vi "GET Log Ref.vi"(8 "error in (no error)":errorcluster) -> (0 "error out":errorcluster, 3 "LogsAbstract out":refnum<class "LogsAbstract.lvclass">)   [LabVIEW 2019, in "LogsAbstract.lvlib" / "LogsAbstract.lvclass"]
uses:
  LogsAbstract.lvclass
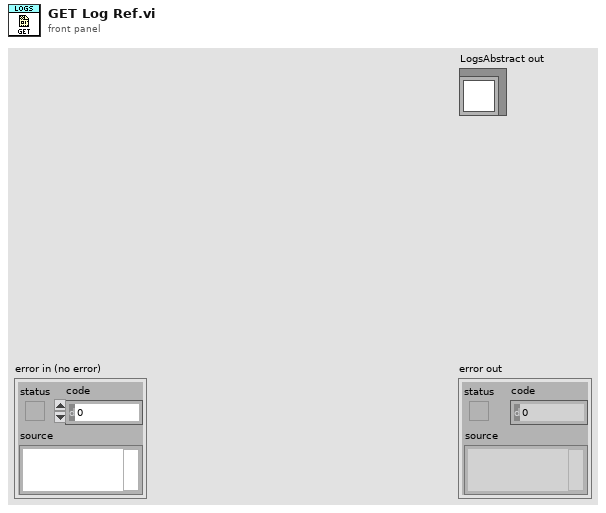
[diagram p1: front panel]
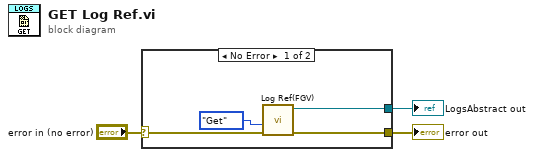
[diagram p0: block diagram]
diagram:
  n1 = case shown="No Error" "error in (no error)" {
    selector: "error in (no error)" -> [w6 w8]
    tunnel: [w5 w8] -> w2
    tunnel: [w7 _] -> w1
    frame No Error {
      n2 = call "Log Ref(FGV).vi"("Error In"=w6, "State"=enum16{"Get", "Set"}."Get") -> ("Error Out"=w5:errorcluster, "EventLog Out"=w7:refnum<class "LogsAbstract.lvclass">)  [unwired: 8 in]
    }
    frame Error {
    }
  }
  "error out" <- w2
  "LogsAbstract out" <- w1
